vi "Analyze Ringdowns.vi"(4 "CellData":T2={"CalType"=enum."LRS", "ErrorCallOn"=FALSE, "lambda (nm)"=0.0, "opticTimeConst"=0.0}, 6 "Filter?":bool, 7 "#_shots":i32=5, 8 "error in":errorcluster, 9 "dt":sgl=1.0, 10 "P":sgl, 11 "CRDS Cell Data in":refnum<class "CRDS Cell Data.lvclass">) -> (0 "error out":errorcluster, 2 "extCr":sgl, 3 "CRDS Cell Data out":refnum<class "CRDS Cell Data.lvclass">)   [LabVIEW 2011]
uses:
  <vilib>/Analysis/NI_AALBase.lvlib
  Reusable/General/Atmospheric/Atmospheric Constants.vi
  CRDS Cell Data.lvclass
  Main Class/Controls/Get Tau Method.ctl
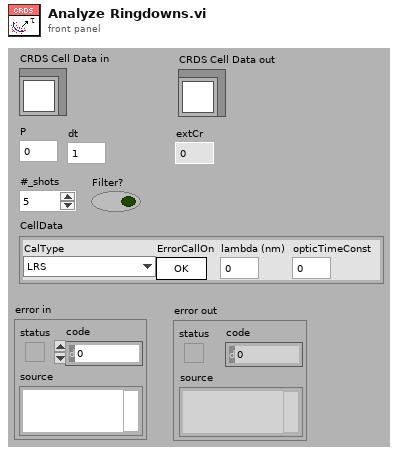
[diagram p1: front panel]
types:
  T1 = typedef "Get Tau Method.ctl" = enum8{"DFT-1", "DFT-5", "LRS"}
  T2 = cluster{"CalType":T1, "ErrorCallOn":bool, "lambda (nm)":dbl, "opticTimeConst":dbl}
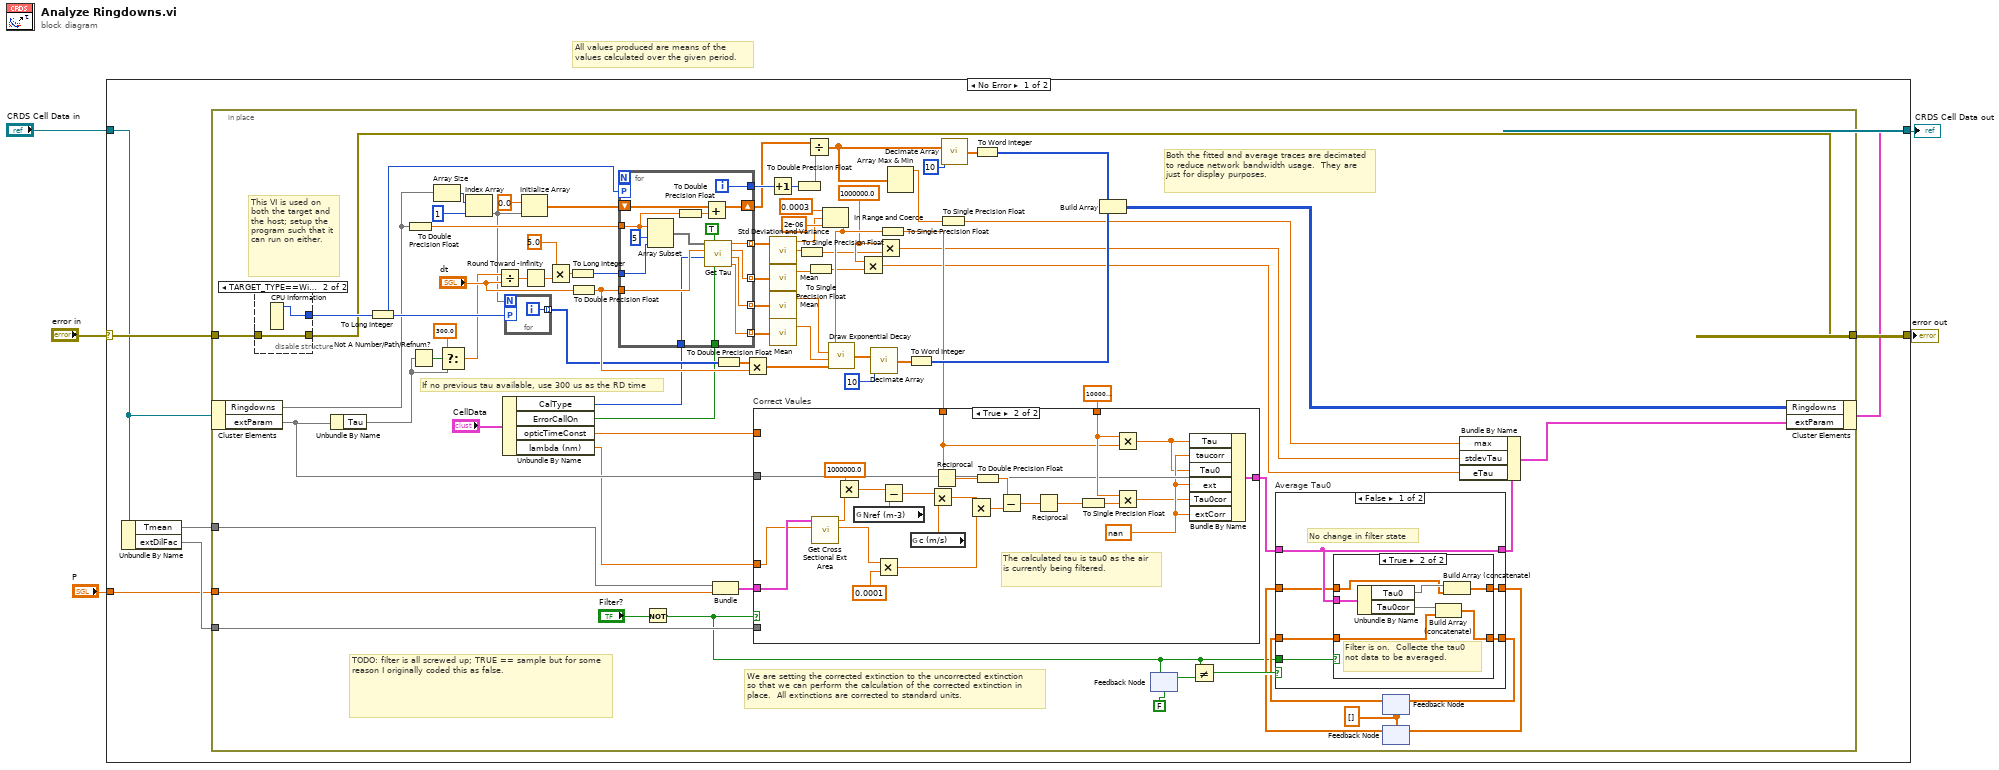
[diagram p0: block diagram]
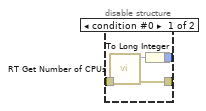
[diagram p2: hidden frame]
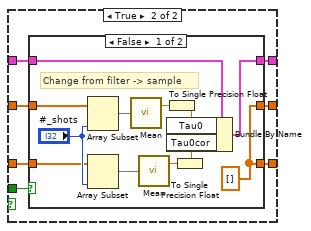
[diagram p4: hidden frame]
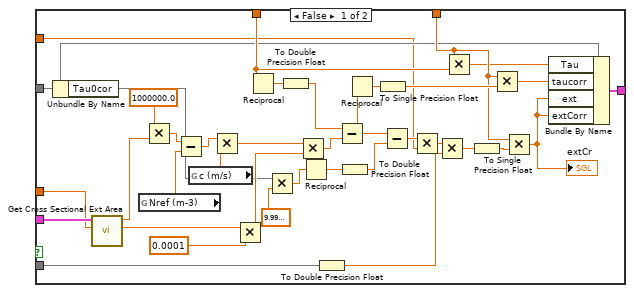
[diagram p6: hidden frame]
diagram:
  # "All values produced are means of the values calculated over the given period."
  n1 = case shown="No Error" "error in" {
    selector: "error in" -> [w12 w218]
    tunnel: [w8 w218] -> w4
    tunnel: [w11 w217] -> w2
    tunnel: "CRDS Cell Data in" -> [w6 w217]
    tunnel: "P" -> [w7 _]
    frame No Error {
      n2 = Unbundle By Name(w6) -> ("Tmean"=w9, "extDilFac"=w10)
      n3 = in-place {
        in-place-border: w12 -> [w19]
        in-place-border: w10 -> [w44]
        in-place-border: w9 -> [w43]
        in-place-border: [w18] -> w8
        in-place-border: w7 -> [w20]
        w38 = sgl[] []
        w81 = sgl 1000000.0
        # "This VI is used on both the target and the host; setup the program such that it can run on either."
        # "If no previous tau available, use 300 us as the RD time"
        # "Both the fitted and average traces are decimated to reduce network bandwidth usage.  They are just for display purposes."
        # "TODO: filter is all screwed up; TRUE == sample but for some reason I originally coded this as false."
        # "We are setting the corrected extinction to the uncorrected extinction so that we can perform the calculation of the corrected extinction in place.  All extinctions are corrected to standard units."
        n4 = in-place-cluster #1(w6) -> ("Ringdowns"=w52, "extParam"=w47)
        n5 = disable-structure shown="TARGET_TYPE==Windows" {
          disable-tunnel: [w98 w100] -> w25
          disable-tunnel: w19 -> [w96 w99]
          disable-tunnel: [w95 w99] -> w18
          frame condition #0 {
            n6 = call <vilib>:"RT Get Number of CPUs.vi"("error in (no error)"=w96) -> ("error out"=w95:errorcluster, "# of CPUs"=w97:u32)  [unwired: 9 in]
            n7 = To Long Integer(number=w97) -> (32bit integer=w98:i32)
          }
          frame condition #1 (active) {
            n8 = CPU Information() -> (4:w100:i32)  [unwired: 3 out]
          }
        }
        n9 = Unbundle By Name(w47) -> ("Tau"=w23)
        n10 = To Long Integer(number=w25) -> (32bit integer=w84:i32)
        n11 = To Double Precision Float(number=w52) -> (double precision float=w91:dbl)
        n12 = Not A Number/Path/Refnum?(number/path/refnum=w23) -> (NaN/Path/Refnum?=w24:bool)
        n13 = Array Size(array=w52) -> (size(s)=w68:i32)
        n14 = Select(t=sgl 300.0, s=w24, f=w23) -> (s? t:f=w21:sgl)
        n15 = Index Array(array=w68, index=1) -> (element=w14)
        n16 = Divide(x=w21, y="dt") -> (x/y=w64:sgl)
        n17 = Unbundle By Name("CellData") -> ("CalType"=w31:T1, "ErrorCallOn"=w30:bool, "opticTimeConst"=w28:dbl, "lambda (nm)"=w29:dbl)
        n18 = for {
          N: w14 -> [_]
          tunnel: [w216] -> w72 mode=indexing
          workers-P: w84 -> [_]
          i -> [w216]
        }
        n19 = Initialize Array(0.0 ("element"), w14) -> (w57:dbl[])
        n20 = Round Toward -Infinity(1:w64) -> (0:w76:sgl)
        n21 = Multiply(x=sgl 5.0 ("y"), y=w76) -> (x*y=w82:sgl)
        n22 = To Long Integer(number=w82) -> (32bit integer=w15:i32)
        n23 = To Double Precision Float(number="dt") -> (double precision float=w92:dbl)
        n24 = for {
          tunnel: [w215] -> w13 mode=indexing
          tunnel: w91 -> [w201]
          tunnel: [w214] -> w53 mode=indexing
          tunnel: [w213] -> w54 mode=indexing
          tunnel: [w212] -> w55 mode=indexing
          shift-right: [w211] -> w58
          shift-left: w57 -> [w209]
          tunnel: w92 -> [w210]
          tunnel: [w206] -> w70
          tunnel: w15 -> [w205]
          workers-P: w84 -> [_]
          tunnel: w31 -> [w203]
          tunnel: w30 -> [w202]
          i -> [w206]
          n25 = Array Subset(array=w201, index=5, length=w205) -> (w200:void[])
          n26 = To Double Precision Float(number=w201) -> (double precision float=w204:dbl)
          n27 = Add(x=w209, y=w204) -> (x+y=w211:dbl[])
          n28 = call "Get Tau.vi"("ErrorCallOn"=w202, "init"=TRUE, "CalType"=w203, "Dt"=w210, "X"=w200) -> ("B"=w212:dbl, "A"=w213:dbl, "e_tau"=w214:dbl, "tau"=w215:dbl)  [unwired: 2 in, 1 out]
        }
        n29 = Not(x="Filter?") -> (.not. x?=w16:bool)
        n30 = Bundle("Tmean"=w43, "P"=w20) -> (w87:cluster{"Tmean":void, "P":sgl})  [unwired: 1 in]
        n31 = To Double Precision Float(number=w72) -> (double precision float=w71:dbl[])
        n32 = Multiply(x=w71, y=w92) -> (x*y=w61:dbl[])
        n33 = Increment(x=w70) -> (x+1=w78:i32)
        n34 = call <vilib>:"Std Deviation and Variance.vi"("X"=w13) -> ("mean"=w65:dbl, "standard deviation"=w74:dbl)  [unwired: 1 in, 1 out]
        n35 = call <vilib>:"Mean.vi"("X"=w53) -> ("mean"=w73:dbl)  [unwired: 1 out]
        n36 = call <vilib>:"Mean.vi"("X"=w54) -> ("mean"=w59:dbl)  [unwired: 1 out]
        n37 = call <vilib>:"Mean.vi"("X"=w55) -> ("mean"=w60:dbl)  [unwired: 1 out]
        n38 = To Double Precision Float(number=w78) -> (double precision float=w77:dbl)
        n39 = To Single Precision Float(number=w74) -> (single precision float=w79:sgl)
        n40 = Divide ("mean")(x=w58, y=w77) -> (x/y=w27:dbl[])
        n41 = To Single Precision Float(number=w73) -> (single precision float=w80:sgl)
        n42 = In Range and Coerce(upper limit=0.0003, x=w65, lower limit=2e-06) -> (coerced(x)=w83:dbl)  [unwired: 1 out]
        n43 = call "Draw Exponential Decay.vi"("time"=w61, "B"=w60, "A"=w59, "tau"=w83) -> ("ExponentialOut"=w62:dbl[])
        n44 = Multiply(x=w81, y=w80) -> (x*y=w48:sgl)
        n45 = call "Decimate Array.vi"("ArrayIn"=w62, "n"=10) -> ("ArrayOut"=w88:dbl[])  [unwired: 13 in]
        n46 = Multiply(x=w81, y=w79) -> (x*y=w49:sgl)
        n47 = To Single Precision Float(number=w83) -> (single precision float=w86:sgl)
        n48 = case "Correct Vaules" shown="True" w16 {
          tunnel: w86 -> [w149 w181]
          tunnel: w87 -> [w174 w199]
          tunnel: w44 -> [w140 _]
          tunnel: sgl 1000000.0 -> [w158 w184]
          tunnel: w47 -> [w146 w180]
          tunnel: [w143 w176] -> w36
          tunnel: w29 -> [w142 w175]
          tunnel: w28 -> [w141 _]
          frame False {
            n49 = Unbundle By Name(w146) -> ("Tau0cor"=w147)
            n50 = call "Get Cross Sectional Ext Area.vi"("l (nm)"=w142, "thermoCond"=w174) -> ("CAext (cm2)"=w170:dbl, "M"=w167:dbl)  [unwired: 8 in]
            n51 = global read "Atmospheric Constants.vi" "Nref (m-3)"() -> (w164:dbl)
            n52 = Multiply(x=1000000.0 ("y"), y=w167) -> (x*y=w165:dbl)
            n53 = Subtract(x=w165, y=w164) -> (x-y=w163:dbl)
            n54 = global read "Atmospheric Constants.vi" "c (m/s)"() -> (w173:dbl)
            n55 = Multiply(x=w163, y=w173) -> (x*y=w166:dbl)
            n56 = Multiply(x=w170, y=0.0001 ("x")) -> (x*y=w151:dbl)
            n57 = Reciprocal(x=w149) -> (1/x=w155:sgl)
            n58 = Multiply(x=w147, y=sgl 1e-06) -> (x*y=w150:sgl)
            n59 = To Double Precision Float(number=w155) -> (double precision float=w154:dbl)
            n60 = Multiply(x=w166, y=w151) -> (x*y=w162:dbl)
            n61 = Reciprocal(x=w150) -> (1/x=w153:sgl)
            n62 = To Double Precision Float(number=w140) -> (double precision float=w139:dbl)
            n63 = Subtract(x=w154, y=w162) -> (x-y=w161:dbl)
            n64 = To Double Precision Float(number=w153) -> (double precision float=w152:dbl)
            n65 = Reciprocal(x=w161) -> (1/x=w160:dbl)
            n66 = To Single Precision Float(number=w160) -> (single precision float=w159:sgl)
            n67 = Subtract(x=w161, y=w152) -> (x-y=w172:dbl)
            n68 = Multiply(x=w172, y=w141) -> (x*y=w169:dbl)
            n69 = Multiply(x=w169, y=w139) -> (x*y=w157:dbl)
            n70 = Multiply(x=w158, y=w149) -> (x*y=w145:sgl)
            n71 = To Single Precision Float(number=w157) -> (single precision float=w156:sgl)
            n72 = Multiply(x=w158, y=w159) -> (x*y=w144:sgl)
            n73 = Multiply(x=w158, y=w156) -> (x*y=w138:sgl)
            "extCr" <- w138
            n74 = Bundle By Name(cluster=w146, "Tau"=w145, "taucorr"=w144, "ext"=w138, "extCorr"=w138) -> (w143:cluster{})
          }
          frame True {
            w179 = sgl nan
            # "The calculated tau is tau0 as the air is currently being filtered."
            n75 = call "Get Cross Sectional Ext Area.vi"("l (nm)"=w175, "thermoCond"=w199) -> ("CAext (cm2)"=w190:dbl, "M"=w191:dbl)  [unwired: 8 in]
            n76 = Multiply(x=1000000.0 ("y"), y=w191) -> (x*y=w198:dbl)
            n77 = global read "Atmospheric Constants.vi" "Nref (m-3)"() -> (w197:dbl)
            n78 = Multiply(x=w190, y=0.0001 ("x")) -> (x*y=w187:dbl)
            n79 = Subtract(x=w198, y=w197) -> (x-y=w196:dbl)
            n80 = global read "Atmospheric Constants.vi" "c (m/s)"() -> (w195:dbl)
            n81 = Multiply(x=w196, y=w195) -> (x*y=w188:dbl)
            n82 = Reciprocal(x=w181) -> (1/x=w185:sgl)
            n83 = Multiply(x=w188, y=w187) -> (x*y=w194:dbl)
            n84 = To Double Precision Float(number=w185) -> (double precision float=w186:dbl)
            n85 = Subtract(x=w186, y=w194) -> (x-y=w193:dbl)
            n86 = Reciprocal(x=w193) -> (1/x=w182:dbl)
            n87 = To Single Precision Float(number=w182) -> (single precision float=w183:sgl)
            n88 = Multiply(x=w184, y=w181) -> (x*y=w178:sgl)
            n89 = Multiply(x=w184, y=w183) -> (x*y=w177:sgl)
            n90 = Bundle By Name(cluster=w180, "Tau"=w178, "taucorr"=w179, "Tau0"=w178, "ext"=w179, "Tau0cor"=w177, "extCorr"=w179) -> (w176:cluster{})
          }
        }
        n91 = Array Max & Min(array=w27) -> (max value=w94:dbl)  [unwired: 3 out]
        n92 = To Word Integer(number=w88) -> (16bit integer=w90:i16[])
        n93 = To Single Precision Float(number=w94) -> (single precision float=w50:sgl)
        n94 = call "Decimate Array.vi"("ArrayIn"=w27, "n"=10) -> ("ArrayOut"=w26:dbl[])  [unwired: 13 in]
        n95 = To Word Integer(number=w26) -> (16bit integer=w89:i16[])
        n96 = Build Array(w89, w90) -> (w51:i16[][])
        n97 = feedback-in #2(w16) -> ()
        n98 = feedback #2(FALSE) -> (w41:bool)
        n99 = Not Equal?(x=w16, y=w41) -> (x != y?=w42:bool)
        n100 = feedback #3(w38) -> (w39:sgl[])
        n101 = feedback #4(w38) -> (w37:sgl[])
        n102 = case "Average Tau0" shown="False" w42 {
          tunnel: w16 -> [w103 w122]
          tunnel: w36 -> [w106 w121]
          tunnel: [w106 w120] -> w35
          tunnel: w37 -> [w105 w119]
          tunnel: [w104 w118] -> w33
          tunnel: w39 -> [w102 w117]
          tunnel: [w101 w116] -> w34
          frame False {
            # "No change in filter state"
            n103 = case shown="True" w103 {
              tunnel: w106 -> [_ w114]
              tunnel: w105 -> [w108 w113]
              tunnel: [w108 w112] -> w104
              tunnel: w102 -> [w107 w110]
              tunnel: [w107 w109] -> w101
              frame False {
                # "On sample."
              }
              frame True {
                # "Filter is on.  Collecte the tau0 not data to be averaged."
                n104 = Unbundle By Name(w114) -> ("Tau0"=w115, "Tau0cor"=w111)
                n105 = Build Array (concatenate)(w111, w110) -> (w109:sgl[])
                n106 = Build Array (concatenate)(w115, w113) -> (w112:sgl[])
              }
            }
          }
          frame True {
            n107 = case shown="False" w122 {
              tunnel: w121 -> [w134 w137]
              tunnel: [w133 w137] -> w120
              tunnel: w119 -> [w132 w136]
              tunnel: [w129 w136] -> w118
              tunnel: w117 -> [w130 w135]
              tunnel: [w129 w135] -> w116
              frame False {
                w129 = sgl[] []
                # "Change from filter -> sample"
                n108 = Array Subset(array=w132, length="#_shots") -> (w128:sgl[])  [unwired: 1 in]
                n109 = Array Subset(array=w130, length="#_shots") -> (w127:sgl[])  [unwired: 1 in]
                n110 = call <vilib>:"Mean.vi"("X"=w128) -> ("mean"=w126:dbl)  [unwired: 1 out]
                n111 = call <vilib>:"Mean.vi"("X"=w127) -> ("mean"=w124:dbl)  [unwired: 1 out]
                n112 = To Single Precision Float(number=w126) -> (single precision float=w125:sgl)
                n113 = To Single Precision Float(number=w124) -> (single precision float=w123:sgl)
                n114 = Bundle By Name(cluster=w134, "Tau0"=w125, "Tau0cor"=w123) -> (w133:cluster{})
              }
              frame True {
                # "Change from sample -> filter. Do nothing, the matrices have already been zeroed."
              }
            }
          }
        }
        n115 = feedback-in #3(w34) -> ()
        n116 = feedback-in #4(w33) -> ()
        n117 = Bundle By Name(cluster=w35, "max"=w50, "stdevTau"=w49, "eTau"=w48) -> (w46:cluster{})
        n118 = in-place-cluster #1("Ringdowns"=w51, "extParam"=w46) -> (w11:cluster{})
      }
    }
    frame Error {
    }
  }
  "error out" <- w4
  "CRDS Cell Data out" <- w2
